vi "Get Module Reference.vi"(8 "error in":errorcluster, 11 "calling module":T2) -> (0 "error out":errorcluster, 3 "module reference":T1)   [LabVIEW 2017, in "Controller.lvlib"]
uses:
  Controller.lvlib
  Global TypeDefs/Registered Modules.ctl
  Private TypeDefs/Module Reference.ctl
  Private TypeDefs/Module Queues.ctl
  Private TypeDefs/Message Queue Element.ctl
  Private TypeDefs/Messages.ctl
  Private TypeDefs/Module Notifiers.ctl
  Private TypeDefs/Dummy Notifier.ctl
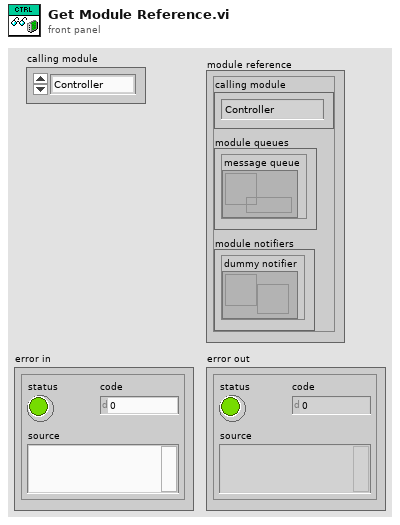
[diagram p1: front panel]
types:
  T1 = typedef "Controller.lvlib/Module Reference.ctl" = cluster{"calling module":T2, "module queues":T3, "module notifiers":T4}
  T2 = typedef "Registered Modules.ctl" = enum16{"Controller", "DAQ", "Error Handler", "Game", "myPAM", "WinHost", "Logger"}
  T3 = typedef "Controller.lvlib/Module Queues.ctl" = cluster{"message queue":refnum<queue>}
  T4 = typedef "Controller.lvlib/Module Notifiers.ctl" = cluster{"dummy notifier":refnum<notifier>}
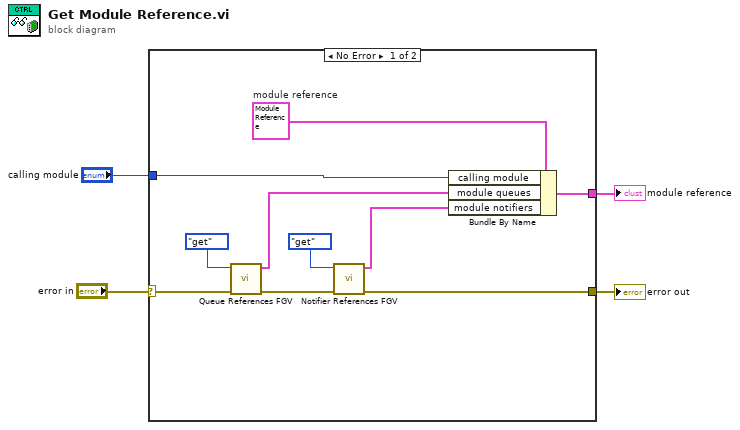
[diagram p0: block diagram]
diagram:
  n1 = case shown="No Error" "error in" {
    selector: "error in" -> [w14 w15]
    tunnel: [w13 w15] -> w3
    tunnel: "calling module" -> [w11 _]
    tunnel: [w8 _] -> w1
    frame No Error {
      w12 = T1 {"calling module"=enum."Controller", "module queues"={"message queue"=refnum}, "module notifiers"={"dummy notifier"=refnum}}  # module reference
      n2 = call "Queue References FGV.vi"("error in"=w14, "function"=enum16{"obtain", "get", "release"}."get") -> ("error out"=w6:errorcluster, "module queues"=w10:T3)  [unwired: 8 in]
      n3 = call "Notifier References FGV.vi"("error in"=w6, "function"=enum16{"obtain", "get", "release"}."get") -> ("error out"=w13:errorcluster, "module notifiers"=w9:T4)  [unwired: 8 in]
      n4 = Bundle By Name(cluster=w12, "calling module"=w11, "module queues"=w10, "module notifiers"=w9) -> (w8:T1)
    }
    frame Error {
    }
  }
  "error out" <- w3
  "module reference" <- w1
